vi "Execute simultaneous move.vi"(8 "error in":errorcluster, 11 "Module ID":i32=-1) -> (0 "error out":errorcluster)   [LabVIEW 2020, in "FCR100.lvlib"]
doc: "Request to execute simultaneous move. Configure simultaneous move beforewards.\n_____\nCreated using DQMH Event Scripter 6.1.0.128."
uses:
  FCR100.lvlib
  Execute simultaneous move Argument--cluster.ctl
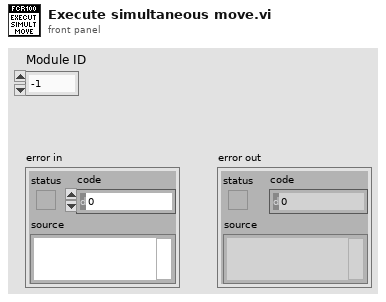
[diagram p1: front panel]
types:
  T1 = typedef "FCR100.lvlib/Execute simultaneous move Argument--cluster.ctl" = cluster{"Module ID":i32, "Boolean":bool}
  T2 = typedef "FCR100.lvlib/Request Events--cluster.ctl" = cluster{"Stop Module":refnum<user-event>, "Show Panel":refnum<user-event>, "Hide Panel":refnum<user-event>, "Show Diagram":refnum<user-event>, "Get Module Execution Status":refnum<user-event>, "Connect with dialog":refnum<user-event>, "Change configuration state":refnum<user-event>, "Change disable state":refnum<user-event>, "Search Home":refnum<user-event>, "Stop movement":refnum<user-event>, "Get state":refnum<user-event>, "Set acceleration":refnum<user-event>, "Get acceleration":refnum<user-event>, "Set velocity":refnum<user-event>, "Get velocity":refnum<user-event>, "Get ETA":refnum<user-event>, "Move absolute":refnum<user-event>, "Move relative":refnum<user-event>, "Get current position":refnum<user-event>, "Reset controller":refnum<user-event>, "Find instruments":refnum<user-event>, "Connect wihtout dialog":refnum<user-event>, "Disconnect":refnum<user-event>, "Continuously check state":refnum<user-event>, "Stop checking state":refnum<user-event>, "Configure simultaneous move":refnum<user-event>, "Get simultaneous move config":refnum<user-event>, "Execute simultaneous move":refnum<user-event>}
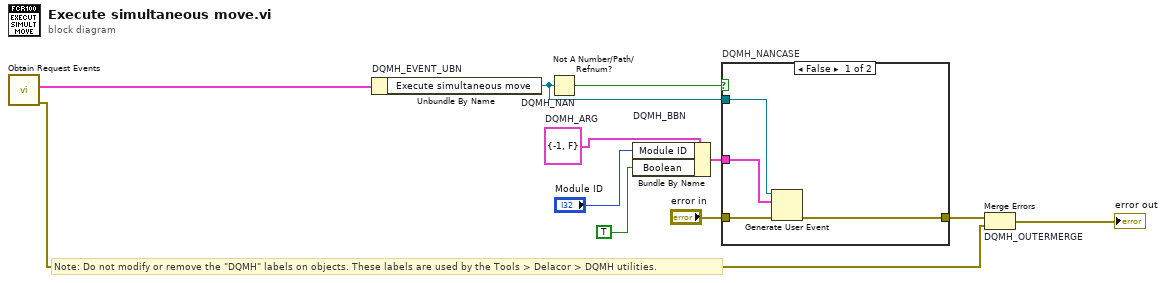
[diagram p0: block diagram]
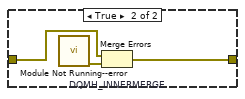
[diagram p2: hidden frame]
diagram:
  w5 = T1 {"Module ID"=-1, "Boolean"=FALSE}  # DQMH_ARG
  # "Note: Do not modify or remove the \"DQMH\" labels on objects. These labels are used by the Tools > Delacor > DQMH utilities."
  n1 = call "Obtain Request Events.vi"() -> ("error out"=w2:errorcluster, "FCR100 Request Events"=w1:T2)  [unwired: 10 in]
  n2 = Unbundle By Name "DQMH_EVENT_UBN"(w1) -> ("Execute simultaneous move"=w7:refnum<user-event>)
  n3 = Not A Number/Path/Refnum? "DQMH_NAN"(number/path/refnum=w7) -> (NaN/Path/Refnum?=w8:bool)
  n4 = Bundle By Name "DQMH_BBN"(cluster=w5, "Module ID"="Module ID", "Boolean"=TRUE) -> (w9:T1)
  n5 = case "DQMH_NANCASE" shown="False" w8 {
    tunnel: "error in" -> [w15 w18]
    tunnel: [w14 w17] -> w6
    tunnel: w7 -> [w13 _]
    tunnel: w9 -> [w12 _]
    frame False {
      n6 = Generate User Event(user event=w13, event data cluster=w12, error in=w15) -> (error out=w14:errorcluster)  [unwired: 1 in, 1 out]
    }
    frame True {
      n7 = call "Module Not Running--error.vi"() -> ("error out"=w16:errorcluster)  [unwired: 11 in]
      n8 = Merge Errors "DQMH_INNERMERGE"(w18, w16) -> (w17:errorcluster)
    }
  }
  n9 = Merge Errors "DQMH_OUTERMERGE"(w6, w2) -> (→"error out":errorcluster)
